vi "PVCAM_StartSeq.vi"(8 "error in (no error)":errorcluster, 10 "buffer":u16[](array[numeric]), 11 "hCam":i16) -> (0 "error out":errorcluster, 2 "return type":i16, 3 "ImageBuf":u16[](array[numeric]))   [LabVIEW 2021]
uses:
  pvcam64.dll
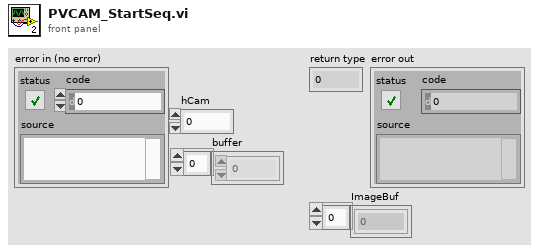
[diagram p1: front panel]
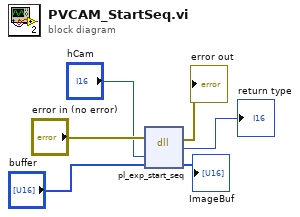
[diagram p0: block diagram]
diagram:
  n1 = dll-call lib="pvcam64.dll" fn="pl_exp_start_seq"(error in="error in (no error)", "hCam"="hCam", "ImageBuf"="buffer") -> (error out=→"error out":errorcluster, "return type"=→"return type":i16, "ImageBuf"=→"ImageBuf":u16[])  [unwired: 3 in, 1 out]
